vi "mini_test_app_serial_gpib_(selectable test mode).vi"() -> ()   [LabVIEW 2015]
doc: "Mini test app for SERIAL RS232 or GPIB communication ports"
uses:
  Type Definitions/Highway_GB_Data.ctl
  Type Definitions/Highway_HP_Data.ctl
  Type Definitions/Highway_Main_Data.ctl
panel:
  out "GB test":dbl(slide) caption="hp time" scale=0.0..3.0 scale format="%#_3g"
  out "HP test":dbl(slide) caption="hp time" scale=0.0..1.0 scale format="%#_3g"
  out "tst time":dbl caption="total test time"
  out "overlap":dbl
  out "2d tst":dbl caption="test time 2"
  out "1st tst":dbl caption="test time 1"
  out "delay":dbl caption="delay time"
  out "mode":string caption="Test mode"
  in  "Stop test":bool
  in  "Start test":bool
  out "HP ID":string="\r\n" caption="Hi-Pot Instrument ID"
  out "GB ID":string="\r\n" caption="GB Instrument ID"
  out "I/F type":string caption="Interface type"
  out "GB tst rslts":string caption="GB test results"
  out "GB tst st":string caption="GB test status"
  out "HP tst rslts":string caption="Results Hi-Pot test"
  in  "Exit Button":bool
  out "HP tst st":string caption="Status Hi-Pot test"
  # "Hi-Pot test"
  # "GB test"
  # "Warning. This app is a proof of concept and has no other purpose, \nit is not intended for production. Use at your own risk."
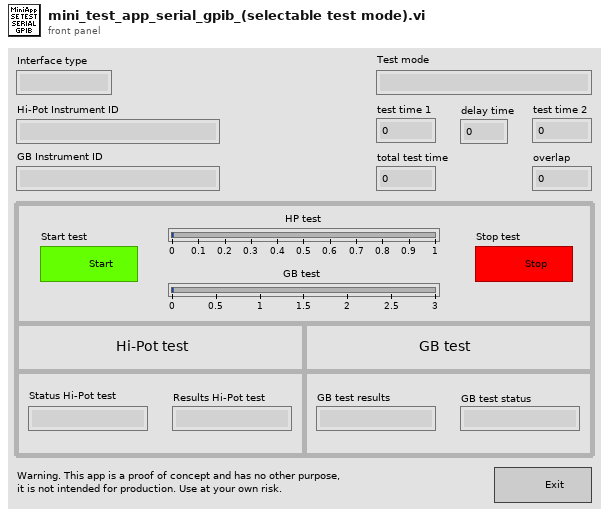
[diagram p1: front panel]
types:
  T1 = typedef "Highway_Main_Data.ctl" = cluster{"Test mode":string, "Delay time":string, "prms":cluster{"1st tst":dbl, "2nd tst":dbl, "overlap":dbl, "tst time":dbl, "tst mod":string, "delay":dbl}}
  T2 = typedef "Highway_HP_Data.ctl" = cluster{"Status HP":string, "Results HP":string}
  T3 = typedef "Highway_GB_Data.ctl" = cluster{"Status GB":string, "Results GB":string}
  T4 = cluster{"Rsrc name for 19572":refnum<visa-resource-name>, "Rsrc name for 19052":refnum<visa-resource-name>, "I/F type":string, "VISA2 Inst ID":string, "VISA1 Inst ID":string}
  T5 = typedef "All Messages Queue.ctl" = cluster{"Main":refnum<queue>, "GB Test":refnum<queue>, "Hi-Pot Test":refnum<queue>}
  T6 = cluster{"1st test":dbl, "2nd test":dbl, "overlap":dbl, "tst time":dbl, "tst mod":string, "delay":dbl}
  T7 = cluster{"1st test":dbl, "2nd test":dbl, "overlap":dbl, "test time":dbl, "test mode":string, "delay":dbl}
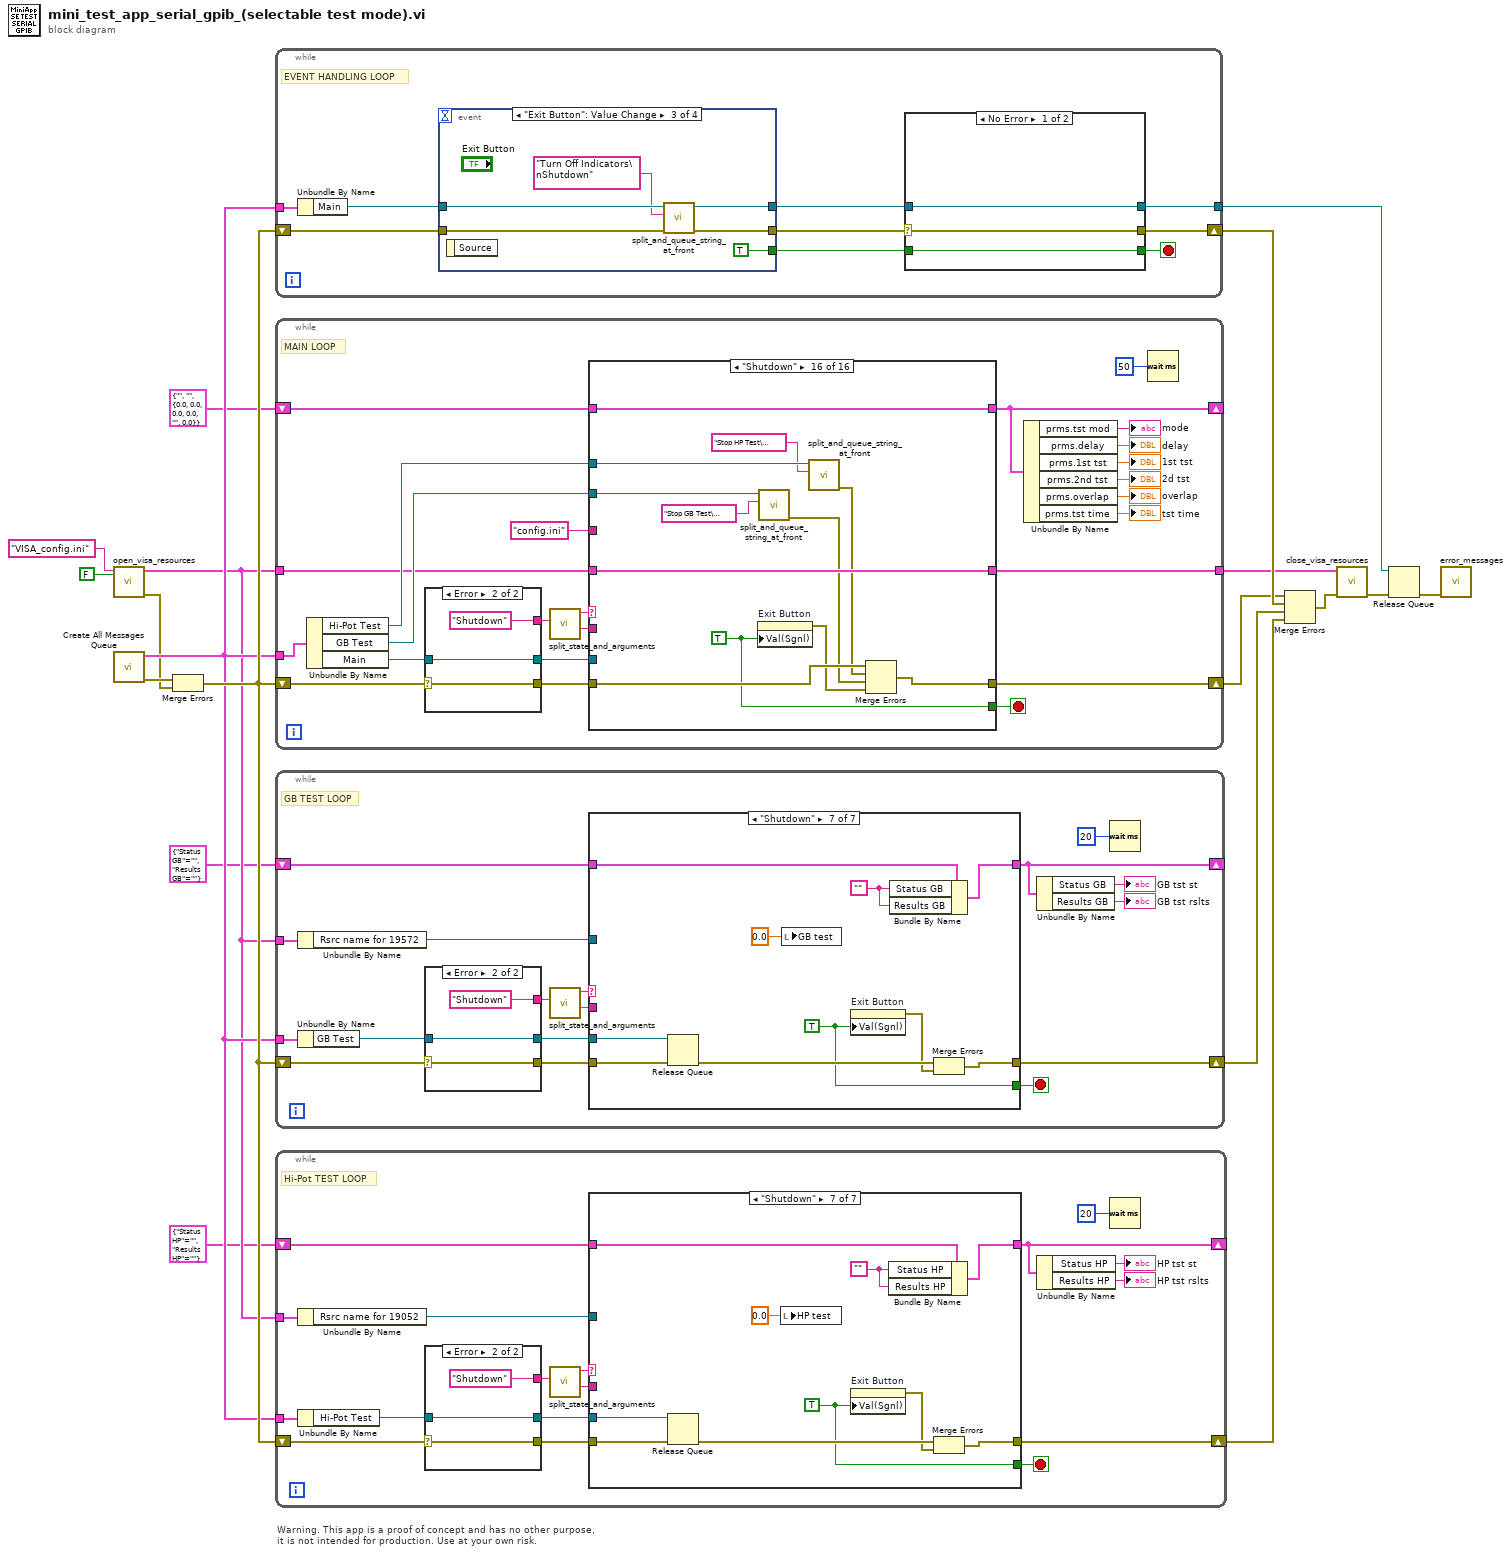
[diagram p0: block diagram]
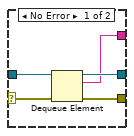
[diagram p2: hidden frame]
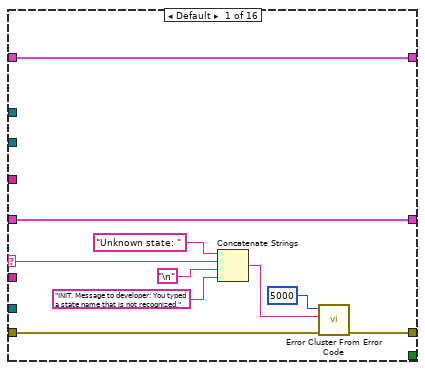
[diagram p3: hidden frame]
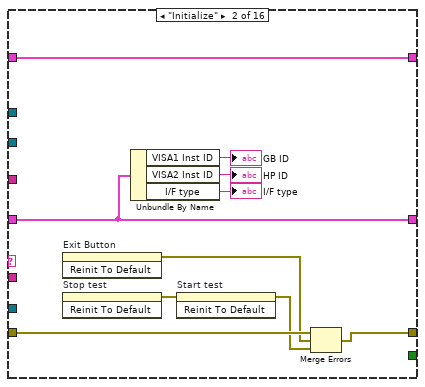
[diagram p4: hidden frame]
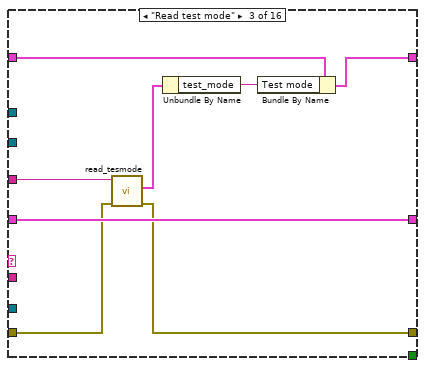
[diagram p5: hidden frame]
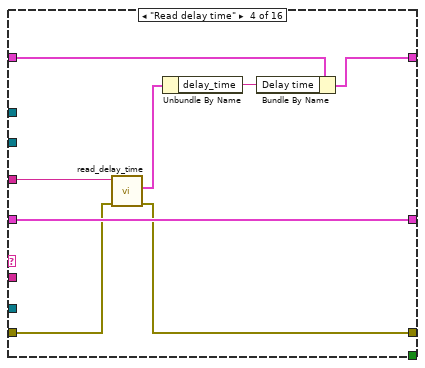
[diagram p6: hidden frame]
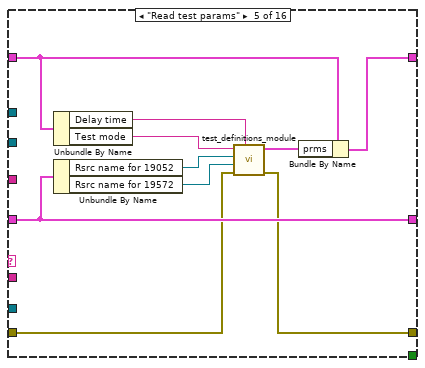
[diagram p7: hidden frame]
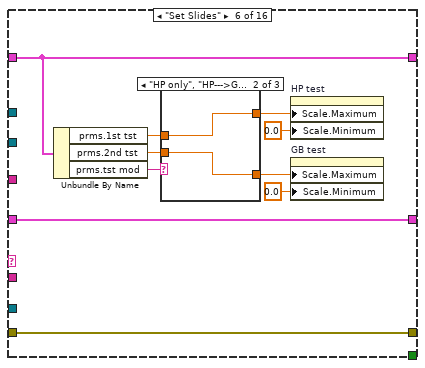
[diagram p8: hidden frame]
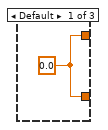
[diagram p9: hidden frame]
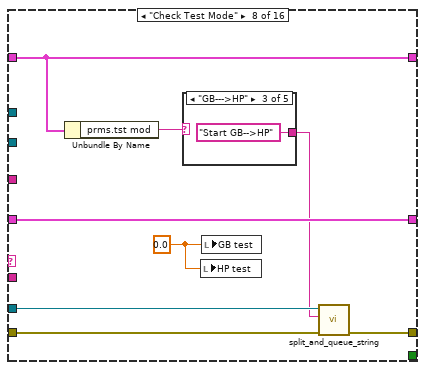
[diagram p12: hidden frame]
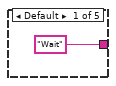
[diagram p13: hidden frame]
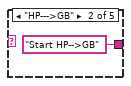
[diagram p14: hidden frame]
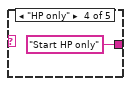
[diagram p15: hidden frame]
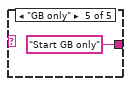
[diagram p16: hidden frame]
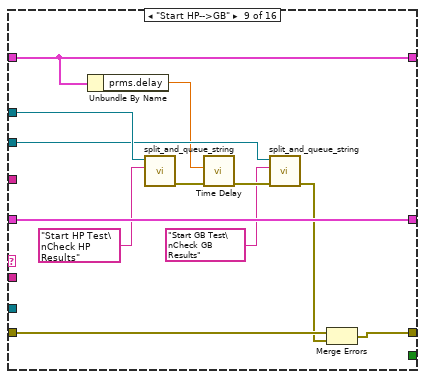
[diagram p17: hidden frame]
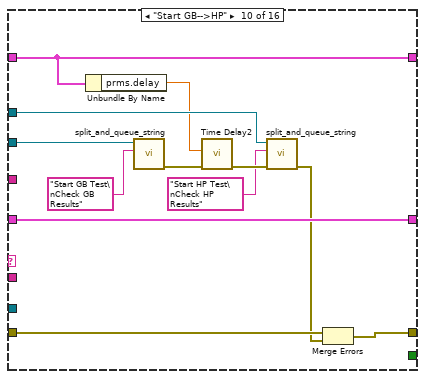
[diagram p18: hidden frame]
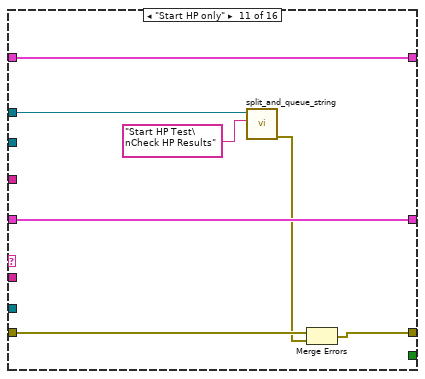
[diagram p19: hidden frame]
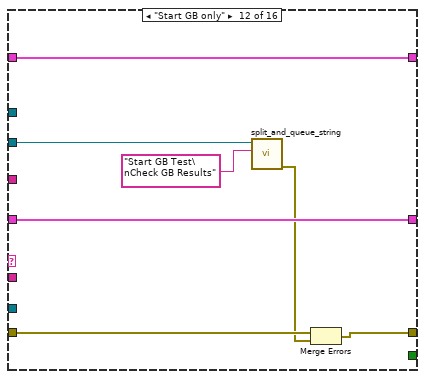
[diagram p20: hidden frame]
diagram:
  # "Warning. This app is a proof of concept and has no other purpose, \nit is not intended for production. Use at your own risk."
  n1 = call "open_visa_resources.vi"("test mode"=FALSE, "config file in"="VISA_config.ini") -> ("error out"=w10:errorcluster, "VISA out"=w9:T4)  [unwired: 8 in]
  n2 = call "Create All Messages Queue.vi"() -> ("error out"=w11:errorcluster, "Messages Queue out"=w18:T5)  [unwired: 10 in]
  n3 = Merge Errors(w11, w10) -> (w19:errorcluster)
  n4 = while {
    shift-right: [w27] -> w14
    shift-left: w19 -> [w28]
    tunnel: w18 -> [w23]
    tunnel: [w20] -> w6
    stop <- w25 stop-if-true
    # "EVENT HANDLING LOOP"
    n5 = Unbundle By Name(w23) -> ("Main"=w22:refnum<queue>)
    n6 = event shown="[2] \"Exit Button\": Value Change" {
      selector: _ -> [_ _ _ _]
      dyn-events: _ -> [_ _ _ _]
      timeout: _ -> [_ _ _ _]
      tunnel: w28 -> [w41 w45 w50 w56]
      tunnel: [w40 w44 w49 w55] -> w24
      tunnel: [_ _ TRUE _] -> w26
      tunnel: w22 -> [w42 w47 w53 w58]
      tunnel: [w38 w43 w48 w54] -> w21
      event "Start test": Value Change {
        n7 = event-data() -> ()  [unwired: 1 in, 1 out]
        n8 = call "split_and_queue_string.vi"("error in (no error)"=w41, "program string"="Check Test Mode", "queue in"=w42) -> ("error out"=w40:errorcluster, "queue out"=w38:refnum<queue>)  [unwired: 7 in]
      }
      event "Stop test": Value Change {
        n9 = event-data() -> ()  [unwired: 1 in, 1 out]
        n10 = call "split_and_queue_string_at_front.vi"("error in (no error)"=w45, "program string"="Stop All Test", "queue in"=w47) -> ("error out"=w44:errorcluster, "queue out"=w43:refnum<queue>)  [unwired: 7 in]
      }
      event "Exit Button": Value Change {
        n11 = event-data() -> ()  [unwired: 1 in, 1 out]
        n12 = call "split_and_queue_string_at_front.vi"("error in (no error)"=w50, "program string"="Turn Off Indicators\nShutdown", "queue in"=w53) -> ("error out"=w49:errorcluster, "queue out"=w48:refnum<queue>)  [unwired: 7 in]
      }
      event Panel Close? {
        n13 = event-data() -> ()  [unwired: 1 in, 1 out]
        n14 = call "split_and_queue_string_at_front.vi"("error in (no error)"=w56, "program string"="Panel Close:Closing App?", "queue in"=w58) -> ("error out"=w55:errorcluster, "queue out"=w54:refnum<queue>)  [unwired: 7 in]
        n15 = event-data("Discard?"=TRUE) -> ()  [unwired: 1 in, 1 out]
      }
    }
    n16 = case shown="No Error" w24 {
      selector: w24 -> [w31 w34]
      tunnel: [w31 w33] -> w27
      tunnel: w26 -> [w30 _]
      tunnel: [w30 TRUE] -> w25
      tunnel: w21 -> [w29 w36]
      tunnel: [w29 w32] -> w20
      frame No Error {
      }
      frame Error {
        n17 = call "split_and_queue_string_at_front.vi"("error in (no error)"=w34, "program string"="Turn Off Indicators\nShutdown", "queue in"=w36) -> ("error out"=w33:errorcluster, "queue out"=w32:refnum<queue>)  [unwired: 7 in]
      }
    }
  }
  n18 = while {
    shift-right: [w81] -> w12
    shift-left: w19 -> [w75]
    tunnel: w9 -> [w60]
    tunnel: [w74] -> w13
    shift-right: [w71] -> _
    shift-left: T1 {"Test mode"="", "Delay time"="", "prms"={"1st tst"=0.0, "2nd tst"=0.0, "overlap"=0.0, "tst time"=0.0, "tst mod"="", "delay"=0.0}} -> [w72]
    tunnel: w18 -> [w61]
    stop <- w77 stop-if-true
    # "MAIN LOOP"
    n19 = Unbundle By Name(w61) -> ("Hi-Pot Test"=w64:refnum<queue>, "GB Test"=w63:refnum<queue>, "Main"=w62:refnum<queue>)
    n20 = case shown="Error" w75 {
      selector: w75 -> [w88 w91]
      tunnel: [w87 w91] -> w82
      tunnel: w62 -> [w84 w90]
      tunnel: [w86 w90] -> w76
      tunnel: [w85 "Shutdown"] -> w79
      frame No Error {
        n21 = Dequeue Element(queue=w84, error in (no error)=w88) -> (queue out=w86:refnum<queue>, element=w85:string, error out=w87:errorcluster)  [unwired: 1 in, 1 out]
      }
      frame Error {
      }
    }
    n22 = call "split_state_and_arguments.vi"("String"=w79) -> ("Arguments"=w78:string, "State"=w80:string)  [unwired: 9 in]
    n23 = case shown="\"Shutdown\"" w80 {
      selector: w80 -> [w97 _ _ _ _ _ _ _ _ _ _ _ _ _ _ _]
      tunnel: [w95 w110 w112 w124 w135 w147 w155 w160 w171 w181 w193 w201 w208 w220 w233 w245] -> w81
      tunnel: w82 -> [w96 w111 w117 w121 w136 w147 w155 w161 w173 w188 w199 w206 w216 w221 w233 w238]
      tunnel: w76 -> [_ _ _ _ _ _ _ w158 _ _ _ _ _ w222 _ _]
      tunnel: w78 -> [_ _ _ _ _ _ _ _ _ _ _ _ _ w224 _ _]
      tunnel: [_ _ _ _ _ _ _ _ _ _ _ _ _ _ _ w234] -> w77
      tunnel: w60 -> [w93 w105 w119 w127 w137 w146 w154 w163 w180 w192 w198 w205 w215 w218 w232 w244]
      tunnel: [w93 w105 w119 w127 w137 w146 w154 w163 w180 w192 w198 w205 w215 w218 w232 w244] -> w74
      tunnel: "config.ini" -> [_ _ w118 w120 _ _ _ _ _ _ _ _ _ _ _ _]
      tunnel: w72 -> [w92 w104 w115 w126 w129 w140 w153 w162 w175 w189 w197 w204 w214 w217 w228 w243]
      tunnel: [w92 w104 w114 w125 w128 w140 w153 w162 w175 w189 w197 w204 w214 w217 w227 w243] -> w71
      tunnel: w64 -> [_ _ _ _ _ _ _ _ w179 w183 w196 _ w213 _ _ w242]
      tunnel: w63 -> [_ _ _ _ _ _ _ _ w178 w184 _ w202 w212 _ _ w240]
      frame Default {
        n24 = Concatenate Strings("Unknown state: " ("string"), w97, "\n", "INIT. Message to developer: You typed a state name that is not recognized.") -> (w99:string)
        n25 = call <vilib>:"Error Cluster From Error Code.vi"("error in (no error)"=w96, "error message (\"\")"=w99, "error code (0)"=5000) -> ("error out"=w95:errorcluster)  [unwired: 6 in]
      }
      frame "Initialize" {
        n26 = invoke on="Exit Button" class="Bool (strict)" method="Reinit To Default"() -> (error out=w109:errorcluster)  [unwired: 3 in, 2 out]
        n27 = invoke on="Stop test" class="Bool" method="Reinit To Default"() -> (error out=w103:errorcluster)  [unwired: 3 in, 2 out]
        n28 = Unbundle By Name(w105) -> ("VISA1 Inst ID"=→"GB ID":string, "VISA2 Inst ID"=→"HP ID":string, "I/F type"=→"I/F type":string)
        n29 = invoke on="Start test" class="Bool" method="Reinit To Default"(error in=w103) -> (error out=w102:errorcluster)  [unwired: 2 in, 2 out]
        n30 = Merge Errors(w111, w109, w102) -> (w110:errorcluster)
      }
      frame "Read test mode" {
        n31 = call "read_tesmode.vi"("error in (no error)"=w117, "config_file_name"=w118) -> ("error out"=w112:errorcluster, "values"=w113:cluster{"test_mode":string})  [unwired: 7 in, 1 out]
        n32 = Unbundle By Name(w113) -> ("test_mode"=w116:string)
        n33 = Bundle By Name(cluster=w115, "Test mode"=w116) -> (w114:T1)
      }
      frame "Read delay time" {
        n34 = call "read_delay_time.vi"("error in (no error)"=w121, "config_file_name"=w120) -> ("error out"=w124:errorcluster, "values"=w122:cluster{"delay_time":string})  [unwired: 7 in, 1 out]
        n35 = Unbundle By Name(w122) -> ("delay_time"=w123:string)
        n36 = Bundle By Name(cluster=w126, "Delay time"=w123) -> (w125:T1)
      }
      frame "Read test params" {
        n37 = Unbundle By Name(w129) -> ("Delay time"=w133:string, "Test mode"=w134:string)
        n38 = Unbundle By Name(w137) -> ("Rsrc name for 19052"=w132:refnum<visa-resource-name>, "Rsrc name for 19572"=w131:refnum<visa-resource-name>)
        n39 = call "test_definitions_module.vi"("Delay time"=w133, "error in (no error)"=w136, "VISA resource in 19572"=w131, "VISA resource in 19052"=w132, "Test mode"=w134) -> ("error out"=w135:errorcluster, "Mode parameters"=w130:T7)  [unwired: 5 in]
        n40 = Bundle By Name(cluster=w129, "prms"=w130) -> (w128:T1)
      }
      frame "Set Slides" {
        n41 = Unbundle By Name(w140) -> ("prms.1st tst"=w144:dbl, "prms.2nd tst"=w143:dbl, "prms.tst mod"=w145:string)
        n42 = case shown="\"HP only\", \"HP--->GB\"" w145 {
          tunnel: w144 -> [_ w150 w152]
          tunnel: w143 -> [_ w149 w151]
          tunnel: [w148 w150 w151] -> w142
          tunnel: [w148 w149 w152] -> w141
          frame Default {
            w148 = 0.0
          }
          frame "HP only", "HP--->GB" {
          }
          frame "GB only", "GB--->HP" {
          }
        }
        n43 = property on="HP test" class="Slide (strict)"("Scale.Maximum"=w142, "Scale.Minimum"=0.0 ("Scale.Range:Minimum")) -> ()  [unwired: 2 in, 2 out]
        n44 = property on="GB test" class="Slide (strict)"("Scale.Maximum"=w141, "Scale.Minimum"=0.0 ("Scale.Range:Minimum")) -> ()  [unwired: 2 in, 2 out]
      }
      frame "Wait" {
      }
      frame "Check Test Mode" {
        w156 = 0.0
        n45 = Unbundle By Name(w162) -> ("prms.tst mod"=w159:string)
        n46 = case shown="\"GB--->HP\"" w159 {
          tunnel: ["Wait" "Start HP-->GB" "Start GB-->HP" "Start HP only" "Start GB only"] -> w157
          frame Default {
          }
          frame "HP--->GB" {
          }
          frame "GB--->HP" {
          }
          frame "HP only" {
          }
          frame "GB only" {
          }
        }
        n47 = local write "HP test"(w156) -> ()
        n48 = local write "GB test"(w156) -> ()
        n49 = call "split_and_queue_string.vi"("error in (no error)"=w161, "program string"=w157, "queue in"=w158) -> ("error out"=w160:errorcluster)  [unwired: 7 in, 1 out]
      }
      frame "Start HP-->GB" {
        n50 = Unbundle By Name(w175) -> ("prms.delay"=w174:dbl)
        n51 = call "split_and_queue_string.vi"("program string"="Start HP Test\nCheck HP Results", "queue in"=w179) -> ("error out"=w177:errorcluster)  [unwired: 8 in, 1 out]
        n52 = call "Time Delay"("error in (no error)"=w177, "Delay Time (s)"=w174) -> ("error out"=w176:errorcluster)  [unwired: 9 in]
        n53 = call "split_and_queue_string.vi"("error in (no error)"=w176, "program string"="Start GB Test\nCheck GB Results", "queue in"=w178) -> ("error out"=w170:errorcluster)  [unwired: 7 in, 1 out]
        n54 = Merge Errors(w173, w170) -> (w171:errorcluster)
      }
      frame "Start GB-->HP" {
        n55 = Unbundle By Name(w189) -> ("prms.delay"=w182:dbl)
        n56 = call "split_and_queue_string.vi"("program string"="Start GB Test\nCheck GB Results", "queue in"=w184) -> ("error out"=w191:errorcluster)  [unwired: 8 in, 1 out]
        n57 = call "Time Delay2"("error in (no error)"=w191, "Delay Time (s)"=w182) -> ("error out"=w190:errorcluster)  [unwired: 9 in]
        n58 = call "split_and_queue_string.vi"("error in (no error)"=w190, "program string"="Start HP Test\nCheck HP Results", "queue in"=w183) -> ("error out"=w185:errorcluster)  [unwired: 7 in, 1 out]
        n59 = Merge Errors(w188, w185) -> (w181:errorcluster)
      }
      frame "Start HP only" {
        n60 = call "split_and_queue_string.vi"("program string"="Start HP Test\nCheck HP Results", "queue in"=w196) -> ("error out"=w194:errorcluster)  [unwired: 8 in, 1 out]
        n61 = Merge Errors(w199, w194) -> (w193:errorcluster)
      }
      frame "Start GB only" {
        n62 = call "split_and_queue_string.vi"("program string"="Start GB Test\nCheck GB Results", "queue in"=w202) -> ("error out"=w200:errorcluster)  [unwired: 8 in, 1 out]
        n63 = Merge Errors(w206, w200) -> (w201:errorcluster)
      }
      frame "Stop All Test" {
        n64 = call "split_and_queue_string_at_front.vi"("program string"="Stop GB Test", "queue in"=w212) -> ("error out"=w209:errorcluster)  [unwired: 8 in, 1 out]
        n65 = call "split_and_queue_string_at_front.vi"("program string"="Stop HP Test", "queue in"=w213) -> ("error out"=w207:errorcluster)  [unwired: 8 in, 1 out]
        n66 = Merge Errors(w216, w207, w209) -> (w208:errorcluster)
      }
      frame "Panel Close" {
        n67 = Two Button Dialog(message=w224) -> (T button?=w223:bool)  [unwired: 2 in]
        n68 = case shown="True" w223 {
          tunnel: ["Wait" "Shutdown\nTurn Off Indicators"] -> w219
          frame False {
          }
          frame True {
          }
        }
        n69 = call "split_and_queue_string_at_front.vi"("error in (no error)"=w221, "program string"=w219, "queue in"=w222) -> ("error out"=w220:errorcluster)  [unwired: 7 in, 1 out]
      }
      frame "Turn Off Indicators" {
        w229 = ""
        w231 = ""
        n70 = Bundle By Name(cluster=w228, "Test mode"=w229, "Delay time"=w229, "prms"=T6 {"1st test"=0.0, "2nd test"=0.0, "overlap"=0.0, "tst time"=0.0, "tst mod"="", "delay"=0.0} ("md prms")) -> (w227:T1)
        n71 = local write "I/F type"(w231) -> ()
        n72 = local write "HP ID"(w231) -> ()
        n73 = local write "GB ID"(w231) -> ()
      }
      frame "Shutdown" {
        w234 = TRUE
        n74 = property on="Exit Button" class="Bool (strict)"("Val(Sgnl)"=w234) -> (error out=w237:errorcluster)  [unwired: 2 in, 1 out]
        n75 = call "split_and_queue_string_at_front.vi"("program string"="Stop GB Test\nShutdown", "queue in"=w240) -> ("error out"=w236:errorcluster)  [unwired: 8 in, 1 out]
        n76 = call "split_and_queue_string_at_front.vi"("program string"="Stop HP Test\nShutdown", "queue in"=w242) -> ("error out"=w235:errorcluster)  [unwired: 8 in, 1 out]
        n77 = Merge Errors(w238, w235, w236, w237) -> (w245:errorcluster)
      }
    }
    n78 = Unbundle By Name(w71) -> ("prms.tst mod"=→"mode":string, "prms.delay"=→"delay":dbl, "prms.1st tst"=→"1st tst":dbl, "prms.2nd tst"=→"2d tst":dbl, "prms.overlap"=→"overlap":dbl, "prms.tst time"=→"tst time":dbl)
    n79 = Wait (ms)(milliseconds to wait=u32 50) -> ()  [unwired: 1 out]
  }
  n80 = while {
    shift-right: [w260] -> w2
    shift-left: w19 -> [w254]
    tunnel: w9 -> [w249]
    shift-right: [w252] -> _
    shift-left: T3 {"Status GB"="", "Results GB"=""} -> [w253]
    tunnel: w18 -> [w246]
    stop <- w256 stop-if-true
    # "GB TEST LOOP"
    n81 = Unbundle By Name(w249) -> ("Rsrc name for 19572"=w248:refnum<visa-resource-name>)
    n82 = Unbundle By Name(w246) -> ("GB Test"=w247:refnum<queue>)
    n83 = case shown="Error" w254 {
      selector: w254 -> [w267 w270]
      tunnel: [w266 w270] -> w261
      tunnel: w247 -> [w263 w269]
      tunnel: [w265 w269] -> w255
      tunnel: [w264 "Shutdown"] -> w258
      frame No Error {
        n84 = Dequeue Element(queue=w263, error in (no error)=w267) -> (queue out=w265:refnum<queue>, element=w264:string, error out=w266:errorcluster)  [unwired: 1 in, 1 out]
      }
      frame Error {
      }
    }
    n85 = call "split_state_and_arguments.vi"("String"=w258) -> ("Arguments"=w257:string, "State"=w259:string)  [unwired: 9 in]
    n86 = case shown="\"Shutdown\"" w259 {
      selector: w259 -> [w275 _ _ _ _ _ _]
      tunnel: [w273 w282 w285 w300 w311 w315 w323] -> w260
      tunnel: w261 -> [w274 w281 w290 w303 w312 w316 w321]
      tunnel: w255 -> [_ _ _ w304 _ _ w322]
      tunnel: w257 -> [_ _ _ _ _ _ _]
      tunnel: [_ _ _ _ _ _ w318] -> w256
      tunnel: w248 -> [_ _ w289 w297 w310 w314 _]
      tunnel: w253 -> [w271 w283 w288 w296 w309 w313 w326]
      tunnel: [w271 w283 w287 w295 w308 w313 w325] -> w252
      frame Default {
        n87 = Concatenate Strings("Unknown state: " ("string"), w275, "\n", "GB. Message to developer: You typed a state name that is not recognized.") -> (w277:string)
        n88 = call <vilib>:"Error Cluster From Error Code.vi"("error in (no error)"=w274, "error message (\"\")"=w277, "error code (0)"=5000) -> ("error out"=w273:errorcluster)  [unwired: 6 in]
      }
      frame "Initialize" {
        n89 = local write "GB test"(0.0) -> ()
        n90 = Merge Errors(w281) -> (w282:errorcluster)
      }
      frame "Start GB Test" {
        n91 = call "19572 Series START.vi"("error in (no error)"=w290, "VISA resource in"=w289) -> ("error out"=w291:errorcluster)  [unwired: 8 in, 1 out]
        n92 = Bundle By Name(cluster=w288, "Results GB"="") -> (w287:T3)
        n93 = Merge Errors(w291) -> (w285:errorcluster)
        n94 = call "stop_watch_w_feedback_node1.vi"("Command"=enum16{"Elapsed Time", "Reset"}."Reset") -> ()  [unwired: 10 in, 1 out]
      }
      frame "Check GB Results" {
        n95 = call "19572_Get_STATUS.vi"("error in (no error)"=w303, "VISA resource in"=w297) -> ("error out"=w301:errorcluster, "Status"=w294:string)  [unwired: 7 in, 1 out]
        n96 = Bundle By Name(cluster=w296, "Status GB"=w294) -> (w295:T3)
        n97 = Equal?(x=w294, y="RUNNING") -> (x = y?=w298:bool)
        n98 = case shown="False" w298 {
          tunnel: ["Read GB Results" ("program string") "Check GB Results" ("program string")] -> w299
          frame False {
          }
          frame True {
          }
        }
        n99 = call "stop_watch_w_feedback_node1.vi"("Command"=enum16{"Elapsed Time", "Reset"}."Elapsed Time") -> ("Elapsed Time"=→"GB test":dbl)  [unwired: 10 in]
        n100 = call "split_and_queue_string.vi"("error in (no error)"=w301, "program string"=w299, "queue in"=w304) -> ("error out"=w300:errorcluster)  [unwired: 7 in, 1 out]
      }
      frame "Read GB Results" {
        n101 = call "19572 Get_Result_ALL_JUDGMENT.vi"("error in (no error)"=w312, "VISA resource in"=w310) -> ("error out"=w311:errorcluster, "JUDGMENT"=w307:string)  [unwired: 7 in, 1 out]
        n102 = Bundle By Name(cluster=w309, "Results GB"=w307) -> (w308:T3)
      }
      frame "Stop GB Test" {
        n103 = call "19572 Series STOP.vi"("error in (no error)"=w316, "VISA resource in"=w314) -> ("error out"=w315:errorcluster)  [unwired: 8 in, 1 out]
      }
      frame "Shutdown" {
        w324 = ""
        w318 = TRUE
        n104 = Release Queue(queue=w322, error in (no error)=w321) -> (error out=w320:errorcluster)  [unwired: 1 in, 2 out]
        n105 = local write "GB test"(0.0) -> ()
        n106 = property on="Exit Button" class="Bool (strict)"("Val(Sgnl)"=w318) -> (error out=w319:errorcluster)  [unwired: 2 in, 1 out]
        n107 = Bundle By Name(cluster=w326, "Status GB"=w324, "Results GB"=w324) -> (w325:T3)
        n108 = Merge Errors(w320, w319) -> (w323:errorcluster)
      }
    }
    n109 = Unbundle By Name(w252) -> ("Status GB"=→"GB tst st":string, "Results GB"=→"GB tst rslts":string)
    n110 = Wait (ms)(milliseconds to wait=u32 20) -> ()  [unwired: 1 out]
  }
  n111 = while {
    shift-right: [w341] -> w15
    shift-left: w19 -> [w335]
    tunnel: w9 -> [w330]
    shift-right: [w333] -> _
    shift-left: T2 {"Status HP"="", "Results HP"=""} -> [w334]
    tunnel: w18 -> [w327]
    stop <- w337 stop-if-true
    # "Hi-Pot TEST LOOP"
    n112 = Unbundle By Name(w330) -> ("Rsrc name for 19052"=w329:refnum<visa-resource-name>)
    n113 = Unbundle By Name(w327) -> ("Hi-Pot Test"=w328:refnum<queue>)
    n114 = case shown="Error" w335 {
      selector: w335 -> [w348 w351]
      tunnel: [w347 w351] -> w342
      tunnel: w328 -> [w344 w350]
      tunnel: [w346 w350] -> w336
      tunnel: [w345 "Shutdown"] -> w339
      frame No Error {
        n115 = Dequeue Element(queue=w344, error in (no error)=w348) -> (queue out=w346:refnum<queue>, element=w345:string, error out=w347:errorcluster)  [unwired: 1 in, 1 out]
      }
      frame Error {
      }
    }
    n116 = call "split_state_and_arguments.vi"("String"=w339) -> ("Arguments"=w338:string, "State"=w340:string)  [unwired: 9 in]
    n117 = case shown="\"Shutdown\"" w340 {
      selector: w340 -> [w356 _ _ _ _ _ _]
      tunnel: [w354 w363 w365 w380 w391 w395 w404] -> w341
      tunnel: w342 -> [w355 w362 w370 w383 w392 w396 w403]
      tunnel: w336 -> [_ _ _ w385 _ _ w402]
      tunnel: w338 -> [_ _ _ _ _ _ _]
      tunnel: w329 -> [_ _ w371 w384 w393 w397 _]
      tunnel: [_ _ _ _ _ _ w398] -> w337
      tunnel: w334 -> [w352 w364 w369 w377 w390 w394 w407]
      tunnel: [w352 w364 w368 w376 w389 w394 w406] -> w333
      frame Default {
        n118 = Concatenate Strings("Unknown state: " ("string"), w356, "\n", "HP. Message to developer: You typed a state name that is not recognized.") -> (w358:string)
        n119 = call <vilib>:"Error Cluster From Error Code.vi"("error in (no error)"=w355, "error message (\"\")"=w358, "error code (0)"=5000) -> ("error out"=w354:errorcluster)  [unwired: 6 in]
      }
      frame "Initialize" {
        n120 = local write "HP test"(0.0) -> ()
        n121 = Merge Errors(w362) -> (w363:errorcluster)
      }
      frame "Start HP Test" {
        n122 = call "19052 Series START.vi"("error in (no error)"=w370, "VISA resource in"=w371) -> ("error out"=w372:errorcluster)  [unwired: 8 in, 1 out]
        n123 = Bundle By Name(cluster=w369, "Results HP"="") -> (w368:T2)
        n124 = Merge Errors(w372) -> (w365:errorcluster)
        n125 = call "stop_watch_w_feedback_node2.vi"("Command"=enum16{"Elapsed Time", "Reset"}."Reset") -> ()  [unwired: 10 in, 1 out]
      }
      frame "Check HP Results" {
        n126 = call "19052_Get_STATUS.vi"("error in (no error)"=w383, "VISA resource in"=w384) -> ("error out"=w381:errorcluster, "Status"=w375:string)  [unwired: 7 in, 1 out]
        n127 = Bundle By Name(cluster=w377, "Status HP"=w375) -> (w376:T2)
        n128 = Equal?(x=w375, y="RUNNING") -> (x = y?=w378:bool)
        n129 = case shown="False" w378 {
          tunnel: ["Read HP Results" ("program string") "Check HP Results" ("program string")] -> w379
          frame False {
          }
          frame True {
          }
        }
        n130 = call "stop_watch_w_feedback_node2.vi"("Command"=enum16{"Elapsed Time", "Reset"}."Elapsed Time") -> ("Elapsed Time"=→"HP test":dbl)  [unwired: 10 in]
        n131 = call "split_and_queue_string.vi"("error in (no error)"=w381, "program string"=w379, "queue in"=w385) -> ("error out"=w380:errorcluster)  [unwired: 7 in, 1 out]
      }
      frame "Read HP Results" {
        n132 = call "19052 Get_Result_ALL_JUDGMENT.vi"("error in (no error)"=w392, "VISA resource in"=w393) -> ("error out"=w391:errorcluster, "JUDGMENT"=w388:string)  [unwired: 7 in, 1 out]
        n133 = Bundle By Name(cluster=w390, "Results HP"=w388) -> (w389:T2)
      }
      frame "Stop HP Test" {
        n134 = call "19052 Series STOP.vi"("error in (no error)"=w396, "VISA resource in"=w397) -> ("error out"=w395:errorcluster)  [unwired: 8 in, 1 out]
      }
      frame "Shutdown" {
        w398 = TRUE
        w405 = ""
        n135 = Release Queue(queue=w402, error in (no error)=w403) -> (error out=w401:errorcluster)  [unwired: 1 in, 2 out]
        n136 = local write "HP test"(0.0 ("HP test")) -> ()
        n137 = property on="Exit Button" class="Bool (strict)"("Val(Sgnl)"=w398) -> (error out=w400:errorcluster)  [unwired: 2 in, 1 out]
        n138 = Bundle By Name(cluster=w407, "Status HP"=w405, "Results HP"=w405) -> (w406:T2)
        n139 = Merge Errors(w401, w400) -> (w404:errorcluster)
      }
    }
    n140 = Unbundle By Name(w333) -> ("Status HP"=→"HP tst st":string, "Results HP"=→"HP tst rslts":string)
    n141 = Wait (ms)(milliseconds to wait=u32 20) -> ()  [unwired: 1 out]
  }
  n142 = Merge Errors(w12, w14, w2, w15) -> (w1:errorcluster)
  n143 = call "close_visa_resources.vi"("error in (no error)"=w1, "VISA in"=w13) -> ("error out"=w8:errorcluster)  [unwired: 9 in]
  n144 = Release Queue(queue=w6, error in (no error)=w8) -> (error out=w7:errorcluster)  [unwired: 1 in, 2 out]
  n145 = call "error_messages.vi"("error in (no error)"=w7) -> ()  [unwired: 11 in]
